vi "PMUParseConfig.vi"(6 "SyncOK":bool, 8 "error in (no error)":errorcluster, 9 "PMUDataType":T1, 10 "PacketBodyIn":u8[](array[numeric]) format="%x", 11 "C37.118 PMU.lvclass":refnum<class "C37.118 PMU.lvclass">) -> (0 "error out":errorcluster, 3 "C37.118 PMU.lvclass":refnum<class "C37.118 PMU.lvclass">)   [LabVIEW 2014, in "SensorPlugins.lvlib" / "C37.118 PMU.lvclass"]
uses:
  C37.118 PMU.lvclass
  Typedef/FormatBits.ctl
  Typedef/PMUConfigData.ctl
  PmuBaseClass/Typedef/PMUDataType.ctl
  PmuBaseClass/PmuBase.lvclass
  <vilib>/ErrorRing/Error Ring.xnode
  <vilib>/Utility/error.llb/Error Cluster From Error Code.vi
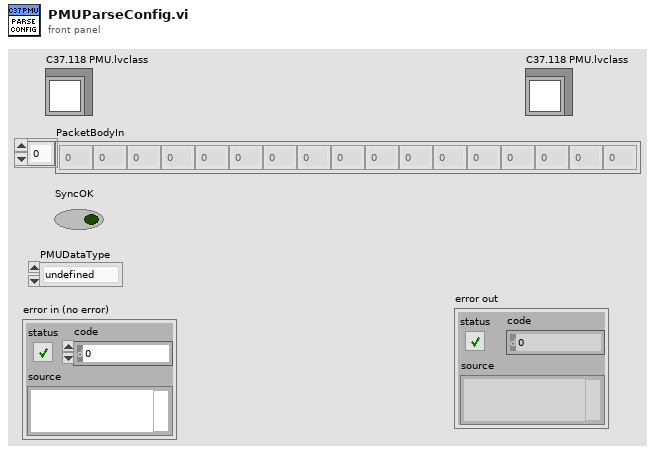
[diagram p1: front panel]
types:
  T1 = typedef "SensorPlugins.lvlib/PmuBase.lvclass/PMUDataType.ctl" = enum16{"undefined", "data", "header", "config 1", "config 2", "config 3", "command"}
  T2 = typedef "SensorPlugins.lvlib/C37.118 PMU.lvclass/FormatBits.ctl" = cluster{"Rect/Polar":bool, "Phasor Int/Float":bool, "Analog Int/Float":bool, "F/ROCOF Int/Float":bool}
  T3 = typedef "SensorPlugins.lvlib/C37.118 PMU.lvclass/PMUConfigData.ctl" = cluster{"TimeBase":u32, "NUM_PMU":u16, "Station Name":string, "IDCODE":u16, "PHRNMR":u16, "ANNMR":u16, "DIGNMR":u16, "FORMAT BITS":T2, "Valid Inputs":u16[], "DigitalStatusMask":u16[], "24bit_PHUNIT":i32[], "24bit_ANUNIT":u32[], "Analog Amplitude Setting":u32[], "Unit (Vor I)":u8[], "ChannelNames":string, "Fs":i16, "SOC ":u32, "FRACSEC":u32, "F0":sgl, "CFGCNT":u16}
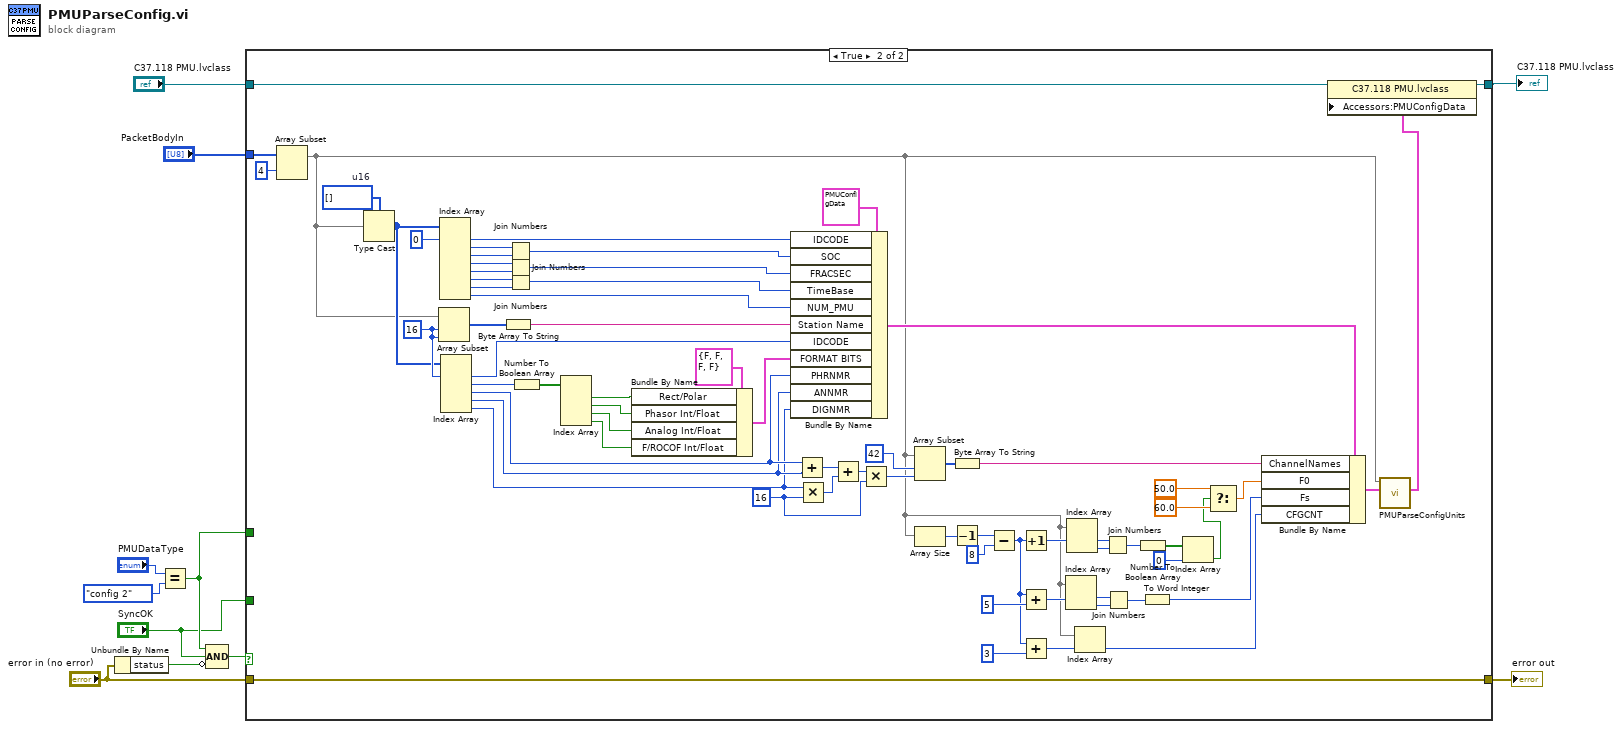
[diagram p0: block diagram]
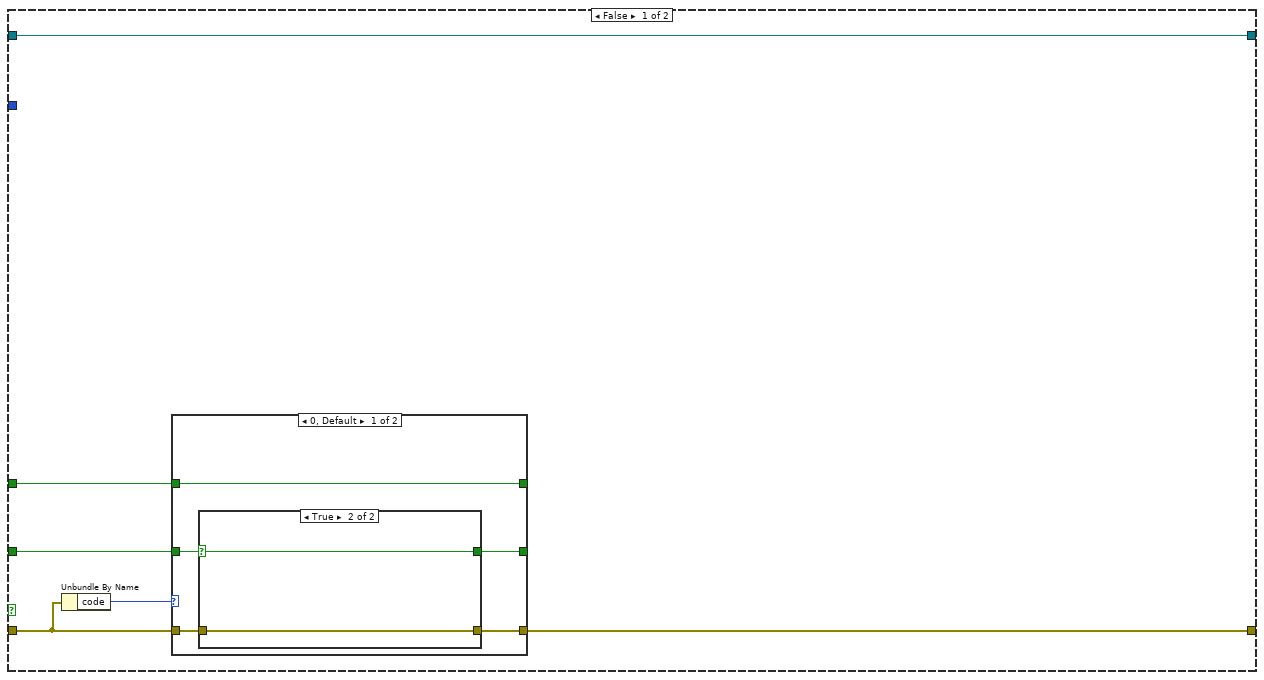
[diagram p2: hidden frame]
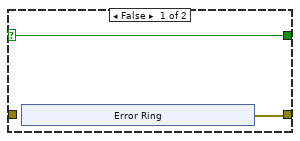
[diagram p3: hidden frame]
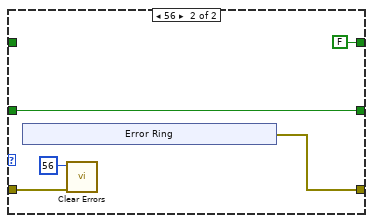
[diagram p4: hidden frame]
diagram:
  n1 = Unbundle By Name("error in (no error)") -> ("status"=w5:bool)
  n2 = Equal?(x="PMUDataType", y=PMUDataType."config 2") -> (x = y?=w2:bool)
  n3 = Compound Arithmetic op=AND(w2, "SyncOK", invert w5) -> (w10:bool)
  n4 = case shown="True" w10 {
    tunnel: "PacketBodyIn" -> [_ w86]
    tunnel: "error in (no error)" -> [w17 w52]
    tunnel: [w15 w52] -> w8
    tunnel: "C37.118 PMU.lvclass" -> [w14 w44]
    tunnel: [w14 w43] -> w3
    tunnel: w2 -> [w13 _]
    tunnel: "SyncOK" -> [w12 _]
    frame False {
      n5 = Unbundle By Name(w17) -> ("code"=w16:i32)
      n6 = case shown="0, Default" w16 {
        tunnel: w13 -> [w22 _]
        tunnel: [w19 w36] -> _
        tunnel: w12 -> [w21 w36]
        tunnel: [w22 FALSE] -> _
        tunnel: w17 -> [w20 w33]
        tunnel: [w18 w32] -> w15
        frame 0, Default {
          n7 = case shown="True" w21 {
            selector: w21 -> [w24 w31]
            tunnel: [w24 w31] -> w19
            tunnel: w20 -> [_ w30]
            tunnel: [w23 w30] -> w18
            frame False {
              n8 = xnode "Error Ring"() -> ("error out"=w23:errorcluster)
            }
            frame True {
            }
          }
        }
        frame 56 {
          n9 = xnode "Error Ring"() -> ("error out"=w32:errorcluster)
          n10 = call <vilib>:"Clear Errors.vi"("error in (no error)"=w33, "specific error code to clear (0: all)"=56) -> ()  [unwired: 4 in, 2 out]
        }
      }
    }
    frame True {
      w77 = u16 16 ("y")
      w96 = 16 ("index")
      w111 = u16[] []  # u16
      n11 = Array Subset(array=w86, index=4) -> (w47:u8[])  [unwired: 1 in]
      n12 = Type Cast(type=w111, x=w47) -> (*(type *) &x=w87:u16[])
      n13 = Array Subset(array=w47, index=w96, length=w96) -> (w85:u8[])
      n14 = Index Array(array=w87, index #1=0 ("index")) -> (element #1=w108:u16, element #2=w107:u16, element #3=w106:u16, element #4=w104:u16, element #5=w103:u16, element #6=w101:u16, element #7=w100:u16, element #8=w98:u16)  [unwired: 7 in]
      n15 = Index Array(array=w87, index #1=w96) -> (element #1=w95:u16, element #2=w94:u16, element #3=w83:u16, element #4=w82:u16, element #5=w81:u16)  [unwired: 4 in]
      n16 = Byte Array To String(unsigned byte array=w85) -> (string=w97:string)
      n17 = Join Numbers(hi=w107, lo=w106) -> ((hi.lo)=w105:u32)
      n18 = Join Numbers(hi=w104, lo=w103) -> ((hi.lo)=w102:u32)
      n19 = Join Numbers(hi=w101, lo=w100) -> ((hi.lo)=w99:u32)
      n20 = Number To Boolean Array(number=w94) -> (Boolean array=w93:bool[])
      n21 = Index Array(array=w93) -> (element #1=w92:bool, element #2=w91:bool, element #3=w90:bool, element #4=w89:bool)  [unwired: 4 in]
      n22 = Bundle By Name(cluster=T2 {"Rect/Polar"=FALSE, "Phasor Int/Float"=FALSE, "Analog Int/Float"=FALSE, "F/ROCOF Int/Float"=FALSE} ("FORMAT BITS"), "Rect/Polar"=w92, "Phasor Int/Float"=w91, "Analog Int/Float"=w90, "F/ROCOF Int/Float"=w89) -> (w88:T2)
      n23 = Bundle By Name(cluster=T3 {"TimeBase"=0, "NUM_PMU"=0, "Station Name"="", "IDCODE"=0, "PHRNMR"=0, "ANNMR"=0, "DIGNMR"=0, "FORMAT BITS"={"Rect/Polar"=FALSE, "Phasor Int/Float"=FALSE, "Analog Int/Float"=FALSE, "F/ROCOF Int/Float"=FALSE}, "Valid Inputs"=[], "DigitalStatusMask"=[], "24bit_PHUNIT"=[], "24bit_ANUNIT"=[], "Analog Amplitude Setting"=[], "Unit (Vor I)"=[], "ChannelNames"="", "Fs"=0, "SOC "=0, "FRACSEC"=0, "F0"=0.0, "CFGCNT"=0} ("PMUConfigData"), "IDCODE"=w108, "SOC"=w105, "FRACSEC"=w102, "TimeBase"=w99, "NUM_PMU"=w98, "Station Name"=w97, "IDCODE"=w95, "FORMAT BITS"=w88, "PHRNMR"=w83, "ANNMR"=w82, "DIGNMR"=w81) -> (w74:T3)
      n24 = Add(x=w83, y=w82) -> (x+y=w80:u16)
      n25 = Multiply(x=w81, y=w77) -> (x*y=w79:u16)
      n26 = Add(x=w80, y=w79) -> (x+y=w78:u16)
      n27 = Multiply(x=w78, y=w77) -> (x*y=w76:u16)
      n28 = Array Subset(array=w47, index=42, length=w76) -> (w73:u8[])
      n29 = Array Size(array=w47) -> (size(s)=w71:i32)
      n30 = Byte Array To String(unsigned byte array=w73) -> (string=w72:string)
      n31 = Decrement(x=w71) -> (x-1=w70:i32)
      n32 = Subtract(x=w70, y=8) -> (x-y=w50:i32)
      n33 = Increment(x=w50) -> (x+1=w68:i32)
      n34 = Add(x=w50, y=5) -> (x+y=w57:i32)
      n35 = Add(x=w50, y=3) -> (x+y=w48:i32)
      n36 = Index Array(array=w47, index #1=w57) -> (element #1=w56:u8, element #2=w55:u8)  [unwired: 1 in]
      n37 = Index Array(array=w47, index #1=w68) -> (element #1=w67:u8, element #2=w66:u8)  [unwired: 1 in]
      n38 = Index Array(array=w47, index=w48) -> (element=w46:u8)
      n39 = Join Numbers(hi=w67, lo=w66) -> ((hi.lo)=w65:u16)
      n40 = Join Numbers(hi=w56, lo=w55) -> ((hi.lo)=w54:u16)
      n41 = Number To Boolean Array(number=w65) -> (Boolean array=w64:bool[])
      n42 = To Word Integer(number=w54) -> (16bit integer=w53:i16)
      n43 = Index Array(array=w64, index=0) -> (element=w59:bool)
      n44 = Select(t=50.0, s=w59, f=60.0) -> (s? t:f=w62:dbl)
      n45 = Bundle By Name(cluster=w74, "ChannelNames"=w72, "F0"=w62, "Fs"=w53, "CFGCNT"=w46) -> (w51:T3)
      n46 = call "PMUParseConfigUnits.vi"("PMUConfig"=w51, "PacketBody"=w47) -> ("PMUConfig"=w42:T3)  [unwired: 8 in, 1 out]
      n47 = property class="C37.118 PMU.lvclass"(reference=w44, "Accessors:PMUConfigData"=w42) -> (reference out=w43:refnum<class "C37.118 PMU.lvclass">)  [unwired: 1 in, 1 out]
    }
  }
  "error out" <- w8
  "C37.118 PMU.lvclass" <- w3
